vi "Option Parser.vi"(0 "Yokogawa WT2X0 in":refnum<class "Yokogawa WT2X0.lvclass">, 1 "ID":string, 2 "THD?":bool, 3 "Number of Cards":dbl, 4 "ID cluster.Model":string, 5 "error in (no error)":errorcluster, 7 "Option":string) -> (14 "Yokogawa WT2X0 out":refnum<class "Yokogawa WT2X0.lvclass">, 19 "error out":errorcluster)   [LabVIEW 2013, in "Universal Power Meter.lvlib" / "Yokogawa WT2X0.lvlib" / "Yokogawa WT2X0.lvclass"]
uses:
  Yokogawa WT2X0.lvclass
  Universal Power Meter class/Universal Power Meter.lvclass
panel:
  out "f":dbl
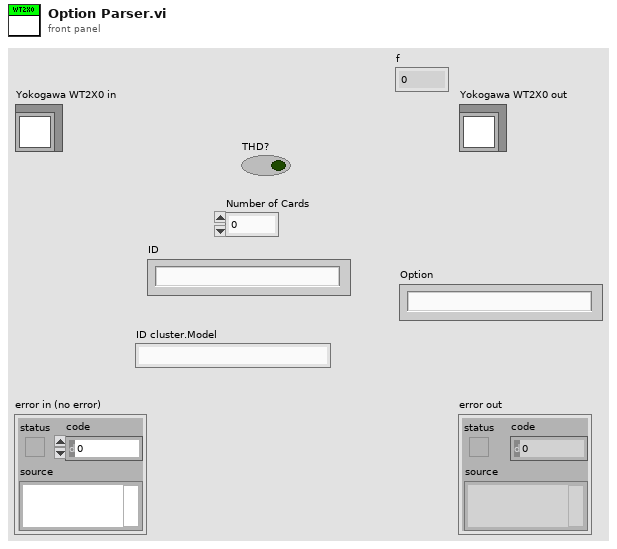
[diagram p1: front panel]
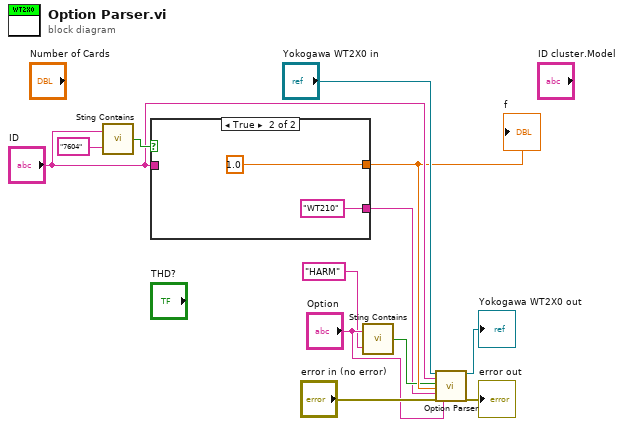
[diagram p0: block diagram]
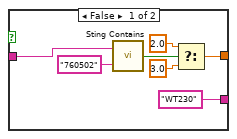
[diagram p2: hidden frame]
diagram:
  n1 = call "Sting Contains.vi"("Expression to evaluate"="7604", "Input String"="ID") -> ("Boolean"=w7:bool)
  n2 = case shown="True" w7 {
    tunnel: [w14 1.0] -> w5
    tunnel: "ID" -> [w19 _]
    tunnel: ["WT230" "WT210"] -> w1
    frame False {
      n3 = call "Sting Contains.vi"("Expression to evaluate"="760502", "Input String"=w19) -> ("Boolean"=w17:bool)
      n4 = Select(t=2.0, s=w17, f=3.0) -> (s? t:f=w14:dbl)
    }
    frame True {
    }
  }
  "f" <- w5
  n5 = call "Sting Contains.vi"("Expression to evaluate"="HARM", "Input String"="Option") -> ("Boolean"=w2:bool)
  n6 = call-parent "Option Parser.vi"("Universal Power Meter in"="Yokogawa WT2X0 in", "ID"="ID", "THD?"=w2, "Number of Cards"=w5, "ID cluster.Model"=w1, "error in (no error)"="error in (no error)", "Option"="Option") -> ("Universal Power Meter out"=→"Yokogawa WT2X0 out":refnum<class "Yokogawa WT2X0.lvclass">, "error out"=→"error out":errorcluster)  [unwired: 11 in]
